vi "L Vread serial.vi"(6 "timoccur":i32, 7 "timeo":i32, 9 "bsize":i32, 10 "buf":u8[](array[numeric])=array[4097 elements], 11 "resourceId":i32) -> (1 "byte read":i32, 2 "buf out":u8[](array[numeric]), 3 "resourceId out":i32, 4 "timoccur out":i32)   [LabVIEW 2010, in "libcommon_serial.lvlib"]
doc: "int LVread_serial(pserial_handle_t h,void*buf,int bsize,int timeo,int*timoccur);"
uses:
  <userlib>/libcommon_serial/libcommon_serial.lvlib
  <userlib>/libcommon_serial/libcommon_serial.so
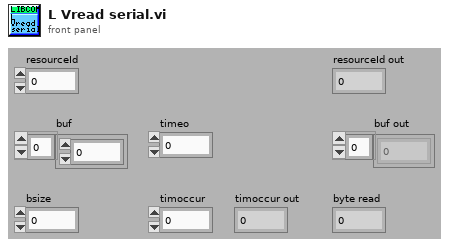
[diagram p1: front panel]
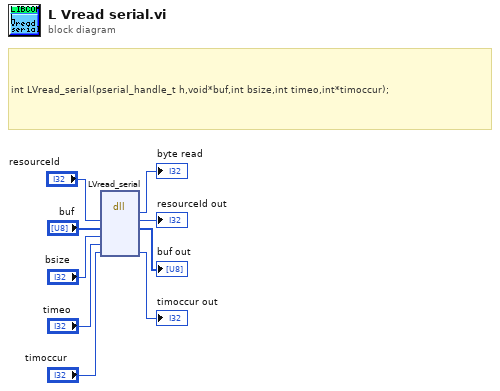
[diagram p0: block diagram]
diagram:
  # "int LVread_serial(pserial_handle_t h,void*buf,int bsize,int timeo,int*timoccur);"
  n1 = dll-call lib="usr/local/natinst/LabVIEW-2010/user.lib/libcommon_serial/libcommon_serial.*" fn="LVread_serial"("resourceId"="resourceId", "buf"="buf", "bsize"="bsize", "timeo"="timeo", "timoccur"="timoccur") -> ("return type"=→"byte read":i32, "resourceId"=→"resourceId out":i32, "buf"=→"buf out":u8[], "timoccur"=→"timoccur out":i32)  [unwired: 5 in, 2 out]
